vi "KE622x -- 2182 -A Check For SCPI Errors.vi"(0 "VISA Resource In":refnum<visa-resource-name>, 11 "error in (no error)":errorcluster) -> (4 "VISA Resource Out (dupl)":refnum<visa-resource-name>, 6 "Error Code":i32[](array[numeric]), 8 "Error Message":string, 15 "error out":errorcluster)   [LabVIEW 2013, in "Keithly user program.lvlib"]
uses:
  Keithly user program.lvlib
panel:
  out "Num Tries":i32
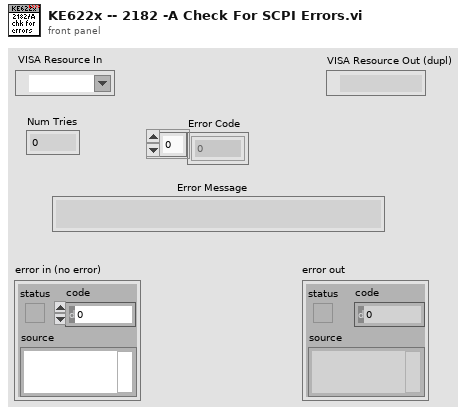
[diagram p1: front panel]
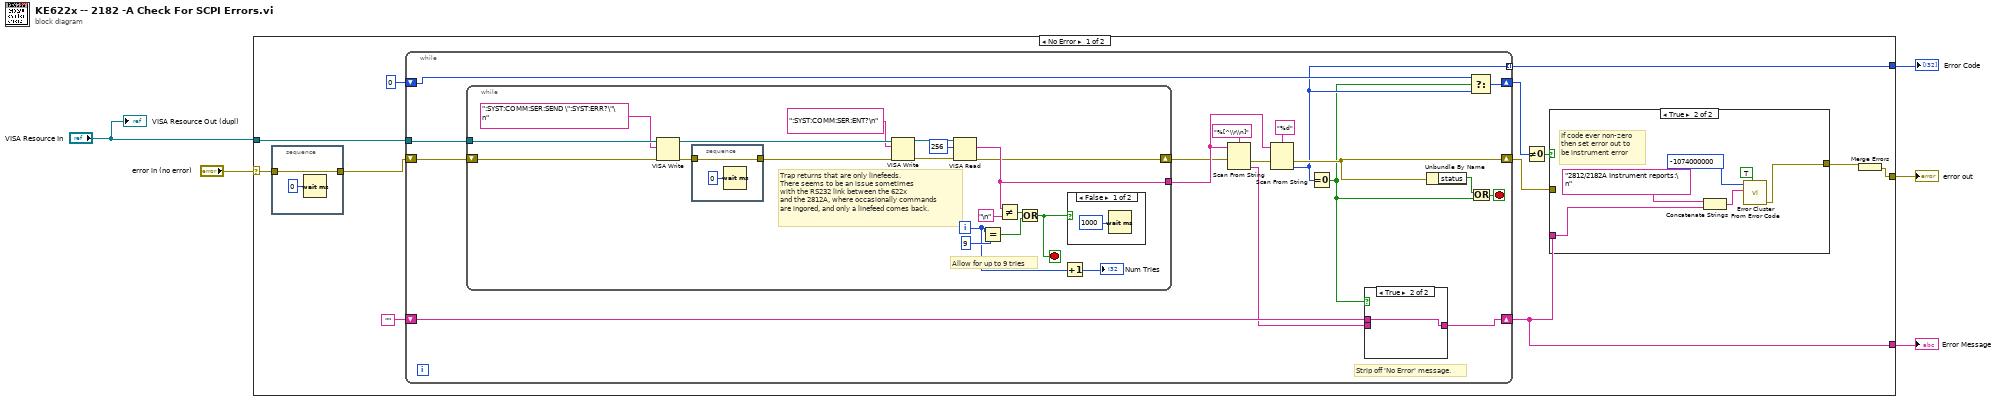
[diagram p0: block diagram]
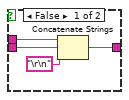
[diagram p4: hidden frame]
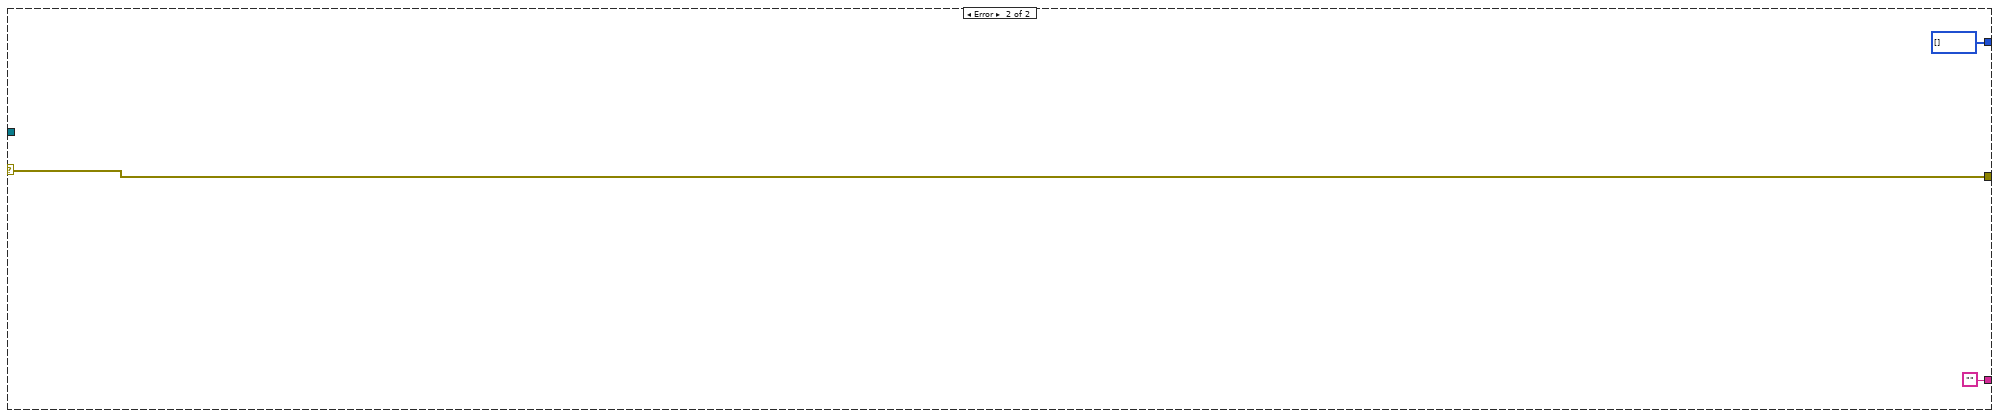
[diagram p5: hidden frame]
diagram:
  n1 = case shown="No Error" "error in (no error)" {
    selector: "error in (no error)" -> [w7 w71]
    tunnel: "VISA Resource In" -> [w17 _]
    tunnel: [w15 w71] -> w5
    tunnel: [w10 ""] -> w4
    tunnel: [w9 i32[] []] -> w3
    frame No Error {
      n2 = stacked-sequence {
        tunnel: w7 -> [w18]
        tunnel: [w18] -> w6
        frame #0 {
          n3 = Wait (ms)(milliseconds to wait=u32 0) -> ()  [unwired: 1 out]
        }
      }
      n4 = while {
        tunnel: w17 -> [w43]
        shift-right: [w37] -> w10
        shift-left: "" -> [w39]
        shift-right: [w35] -> w11
        shift-left: 0 -> [w36]
        shift-right: [w34] -> w8
        shift-left: w6 -> [w29]
        tunnel: [w31] -> w9 mode=indexing
        stop <- w41 stop-if-true
        # "Strip off 'No Error' message."
        n5 = while {
          tunnel: w43 -> [w62]
          tunnel: [w56] -> w28
          shift-right: [w47] -> w27
          shift-left: w29 -> [w61]
          i -> [w45]
          stop <- w46 stop-if-true
          # "Allow for up to 9 tries"
          # "Trap returns that are only linefeeds.\nThere seems to be an issue sometimes\nwith the RS232 link between the 622x\nand the 2812A, where occasionally commands\nare ingored, and only a linefeed comes back."
          n6 = VISA Write(VISA resource name=w62, write buffer=":SYST:COMM:SER:SEND \":SYST:ERR?\"\n" ("Error Query Command"), error in (no error)=w61) -> (VISA resource name out=w59:refnum<visa-resource-name>, error out=w58:errorcluster)  [unwired: 1 out]
          n7 = stacked-sequence {
            tunnel: w58 -> [w64]
            tunnel: [w64] -> w57
            frame #0 {
              n8 = Wait (ms)(milliseconds to wait=u32 0) -> ()  [unwired: 1 out]
            }
          }
          n9 = VISA Write(VISA resource name=w59, write buffer=":SYST:COMM:SER:ENT?\n", error in (no error)=w57) -> (VISA resource name out=w52:refnum<visa-resource-name>, error out=w53:errorcluster)  [unwired: 1 out]
          n10 = VISA Read(VISA resource name=w52, byte count=u32 256, error in (no error)=w53) -> (read buffer=w56:string, error out=w47:errorcluster)  [unwired: 2 out]
          n11 = Equal?(x=w45, y=9) -> (x = y?=w50:bool)
          n12 = Not Equal?(x=w56, y="\n") -> (x != y?=w48:bool)
          n13 = Or(x=w48, y=w50) -> (x .or. y?=w46:bool)
          n14 = Increment(x=w45) -> (x+1=→"Num Tries":i32)
          n15 = case shown="False" w46 {
            frame False {
              n16 = Wait (ms)(milliseconds to wait=u32 1000) -> ()  [unwired: 1 out]
            }
            frame True {
            }
          }
        }
        n17 = Scan From String(format string="%[^\\r\\n]", input string=w28, error in=w27) -> (error out=w33:errorcluster, output 1=w38:string)  [unwired: 1 in, 3 out]
        n18 = Scan From String(format string="%d", input string=w28, error in=w33) -> (error out=w34:errorcluster, output 1=w31:i32)  [unwired: 1 in, 3 out]
        n19 = Equal To 0?(x=w31) -> (x = 0?=w30:bool)
        n20 = case shown="True" w30 {
          tunnel: w39 -> [w69 w70]
          tunnel: w38 -> [w67 _]
          tunnel: [w66 w70] -> w37
          frame False {
            n21 = Concatenate Strings(w69, w67, "\r\n") -> (w66:string)
          }
          frame True {
          }
        }
        n22 = Unbundle By Name(w34) -> ("status"=w32:bool)
        n23 = Select(t=w36, s=w30, f=w31) -> (s? t:f=w35:i32)
        n24 = Or(x=w32, y=w30) -> (x .or. y?=w41:bool)
      }
      n25 = Not Equal To 0?(x=w11) -> (x != 0?=w13:bool)
      n26 = case shown="True" w13 {
        tunnel: w10 -> [_ w25]
        tunnel: [w20 w21] -> w12
        tunnel: w8 -> [w20 _]
        frame False {
        }
        frame True {
          # "If code ever non-zero\nthen set error out to\nbe instrument error"
          n27 = Concatenate Strings("2812/2182A Instrument reports:\n" ("Source"), w25) -> (w22:string)
          n28 = call <vilib>:"Error Cluster From Error Code.vi"("show call chain? (False)"=TRUE, "error message (\"\")"=w22, "error code (0)"=-1074000000 ("Code")) -> ("error out"=w21:errorcluster)  [unwired: 1 in, 5 out]
        }
      }
      n29 = Merge Errors(w12) -> (w15:errorcluster)
    }
    frame Error {
    }
  }
  "error out" <- w5
  "Error Message" <- w4
  "Error Code" <- w3
  "VISA Resource Out (dupl)" <- "VISA Resource In"
